vi "EnumParameterMapping.vi"(8 "Text Ring Control (Using Type Def)":T1=3 items=["Text Value 0", "Text Value 1", "Text Value 2", "Text Value 3", "Text Value 5", "Text Value 6"], 9 "Text Ring (Not Using Type Def)":i32(ring)=78 items=["Text Ring Value - 127"=127, "Text Ring Value - 45"=-45, "Text Ring Value - 78"=78, "Text Ring Value - 11"=-11, "Text Ring Value - 579"=579], 10 "Enum (Using Type Def)":T2=enum."Three", 11 "Enum (Not Using Type Def)":T3(ring)=enum."Value - 2") -> ()   [LabVIEW 2012]
uses:
  EnumTypeDefControl.ctl
  TextRingTypeDefControl.ctl
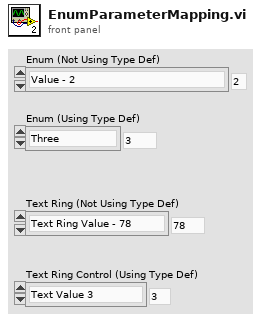
[diagram p1: front panel]
types:
  T1 = typedef "TextRingTypeDefControl.ctl" = u16
  T2 = typedef "EnumTypeDefControl.ctl" = enum8{"Zero", "One", "Two", "Three", "Four", "Five"}
  T3 = enum16{"Value - 0", "Value - 1", "Value - 2", "Value - 3", "Value - 4"}
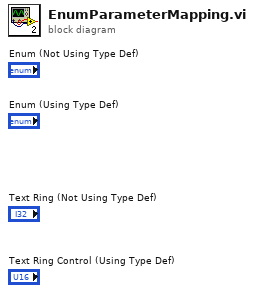
[diagram p0: block diagram]
diagram:
